vi "Illini Hyperloop GUI v2.9.vi"() -> ()   [LabVIEW 2015]
uses:
  <vilib>/ErrorRing/Error Ring.xnode
  BlockDiagramControlEnum.ctl
  <vilib>/robotics/Controls/Attitude Indicator/Attitude Indicator.xctl
  CommunicationStatus.ctl
  StageEnum.ctl
panel:
  in  "Client Closed 2":string="The client VI closed the connection."
  out "Braking Force":dbl
  out "Braking Force Chart":dbl(slide) caption="Braking Force (N)" scale=0.0..10000.0
  out "Current 6":dbl[unit] caption="Current"
  out "Voltage 6":dbl[unit] caption="Voltage"
  out "RPM 6":dbl[unit] caption="RPM"
  out "Current 5":dbl[unit] caption="Current"
  out "Voltage 5":dbl[unit] caption="Voltage"
  out "RPM 5":dbl[unit] caption="RPM"
  out "Current 4":dbl[unit] caption="Current"
  out "Voltage 4":dbl[unit] caption="Voltage"
  out "RPM 4":dbl[unit] caption="RPM"
  out "Current 3":dbl[unit] caption="Current"
  out "Voltage 3":dbl[unit] caption="Voltage"
  out "RPM 3":dbl[unit] caption="RPM"
  out "Current 2":dbl[unit] caption="Current"
  out "Voltage 2":dbl[unit] caption="Voltage"
  out "RPM 2":dbl[unit] caption="RPM"
  out "Current 1":dbl[unit] caption="Current"
  out "Voltage 1":dbl[unit] caption="Voltage"
  out "RPM 1":dbl[unit] caption="RPM"
  out "Flight Time":string
  out "Attitude Indicator":cluster{"Roll":dbl, "Pitch":dbl}(xcontrol)
  out "Yaw":dbl(knob) scale=-20.0..20.0
  out "RPM Gauge 6":dbl(knob) scale=0.0..2000.0
  out "RPM Gauge 5":dbl(knob) scale=0.0..2000.0
  out "RPM Gauge 4":dbl(knob) scale=0.0..2000.0
  out "RPM Gauge 3":dbl(knob) scale=0.0..2000.0
  out "RPM Gauge 2":dbl(knob) scale=0.0..2000.0
  out "RPM Gauge 1":dbl(knob) scale=0.0..2000.0
  out "Cabin Pressure":dbl format="%#.3g"
  out "Cabin Pressure (psi)":dbl(graph)
  out "Stage":T1
  out "Communication Status":T2
  out "Levitation Height":dbl[unit]
  out "Computing:":dbl format="%#.2g"
  out "Low Battery":dbl format="%#.2g"
  out "High Battery:":dbl format="%#.2g"
  out "Battery 3":dbl(slide) scale=0.0..100.0
  out "Battery 2":dbl(slide) scale=0.0..100.0
  out "Battery 1":dbl(slide) scale=0.0..100.0
  out "Z acceleration":dbl
  out "Y acceleration":dbl
  out "X acceleration":dbl
  out "Z velocity":dbl
  out "Y velocity":dbl
  out "X velocity":dbl
  out "Z position":dbl
  out "Y position":dbl
  out "X position":dbl
  out "Position (m)":dbl(slide) scale=0.0..2490.0
  out "Checkmark":u16(ring)
  out "Velocity (m/s)":dbl(graph)
  in  "EMERGENCY BRAKE":bool
  in  "Functional Test Tab Control":T3(tab)
  out "Functional Test A Data":string caption="Data:"
  in  "Functional Test 1":bool caption="Boolean"
  out "Functional Test B Data":string caption="Data:"
  in  "Functional Test 2":bool caption="Boolean"
  out "Functional Test C Data":string caption="Data:"
  in  "Functional Test 3":bool caption="Boolean"
  in  "Functional Test 4":bool caption="Boolean"
  out "Functional Test D Data":string caption="Data:"
  in  "Client Closed":string="The client VI closed the connection."
  out "Data out":string
  out "remote address":string
  out "remote port":u16
  in  "Prepare for Launch":bool caption="Boolean"
  in  "Stop Program":bool
  out "Temp 2:":dbl format="%.2g"
  out "Temp 1:":dbl format="%.2g"
  out "Temperature (K)":dbl[](graph)
  out "Acceleration Chart":dbl(graph)
  # "Illini Hyperloop"
  # "Arx Pax"
  # "Front"
  # "Attitude"
  # "Acceleration (m/s/s)"
  # "Battery Levels (%)"
  # "More battery?????"
  # "Functional Test A: Power Up and Communication"
  # "Functional Test B: Levitation"
  # "Functional Test C: Communication Inside Tube"
  # "Functional Test D: Internal power and Levitation"
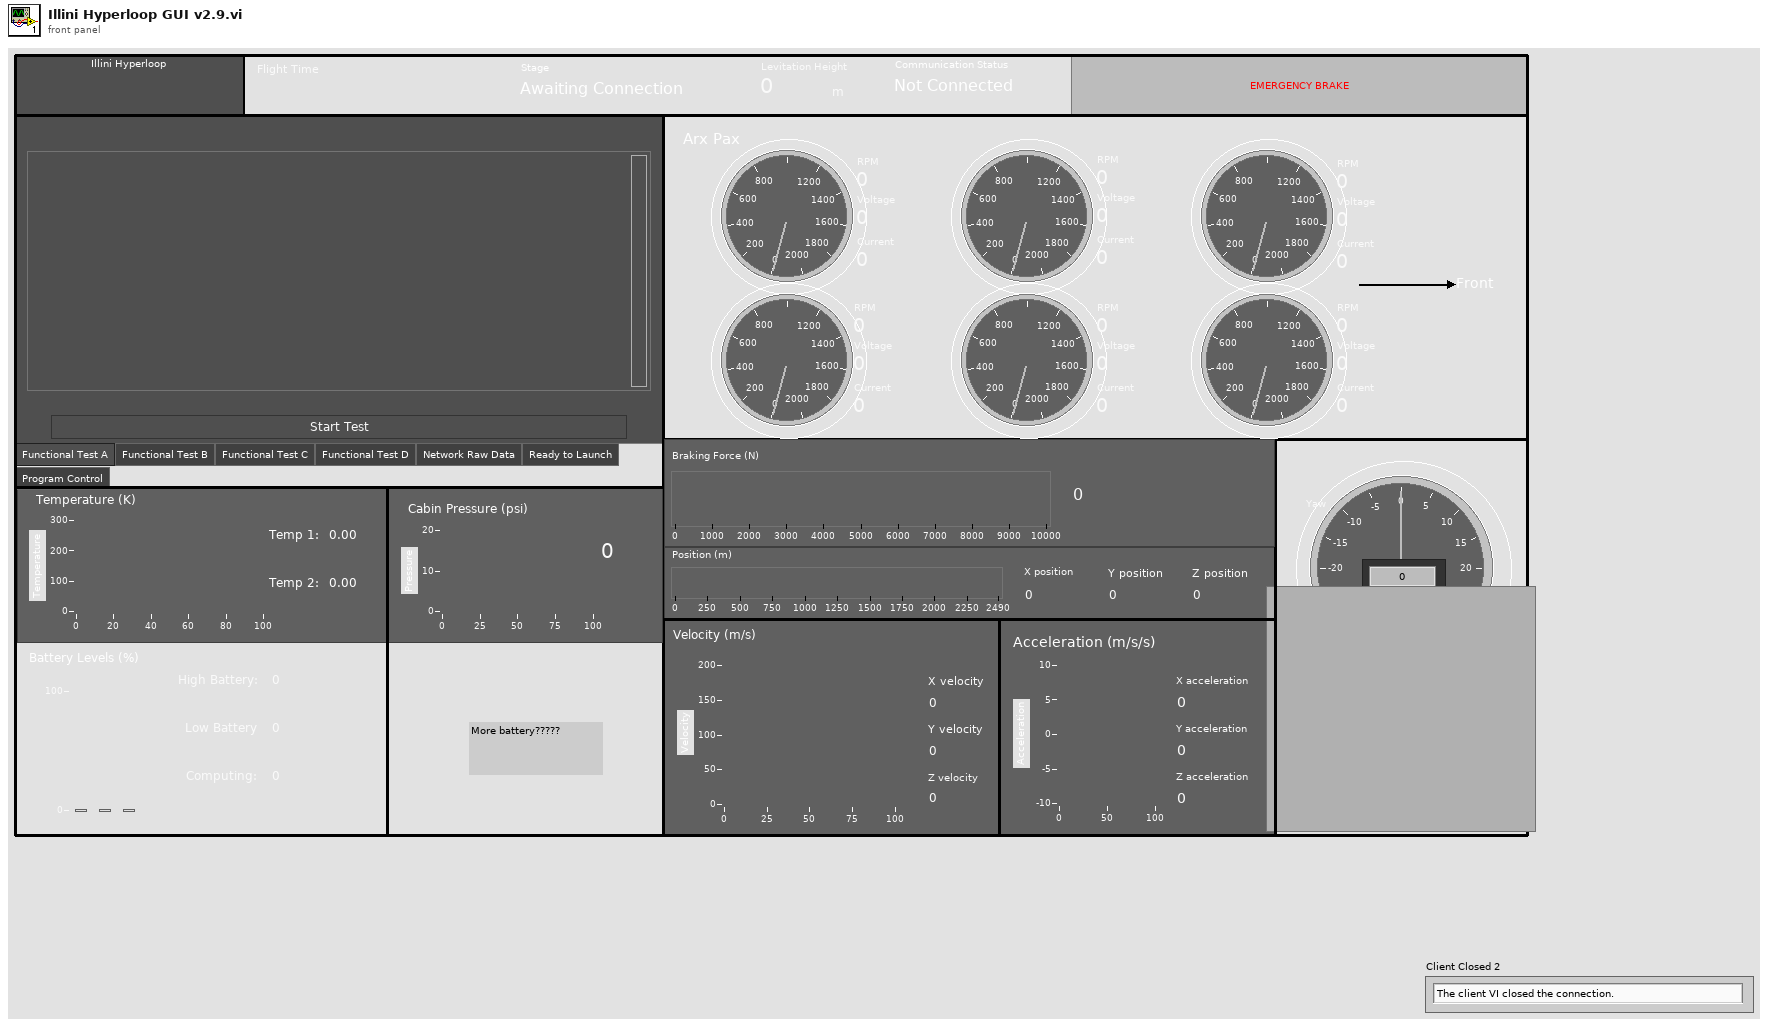
[diagram p1: front panel]
types:
  T1 = typedef "StageEnum.ctl" = enum16{"Awaiting Connection", "TEST Comms", "TEST Lev", "TEST Inside Comms", "TEST Internal Power", "Ready to Launch", "Acceleration", "Coast", "Brake"}
  T2 = typedef "CommunicationStatus.ctl" = enum16{"Not Connected", "Connected", "Disconnected"}
  T3 = enum32{"Functional Test A", "Functional Test B", "Functional Test C", "Functional Test D", "Network Raw Data", "Ready to Launch", "Program Control"}
  T4 = typedef "BlockDiagramControlEnum.ctl" = enum16{"Not Connected", "Disconnected", "Functional Test A", "Functional Test B", "Functional Test C", "Functional Test D", "Flight"}
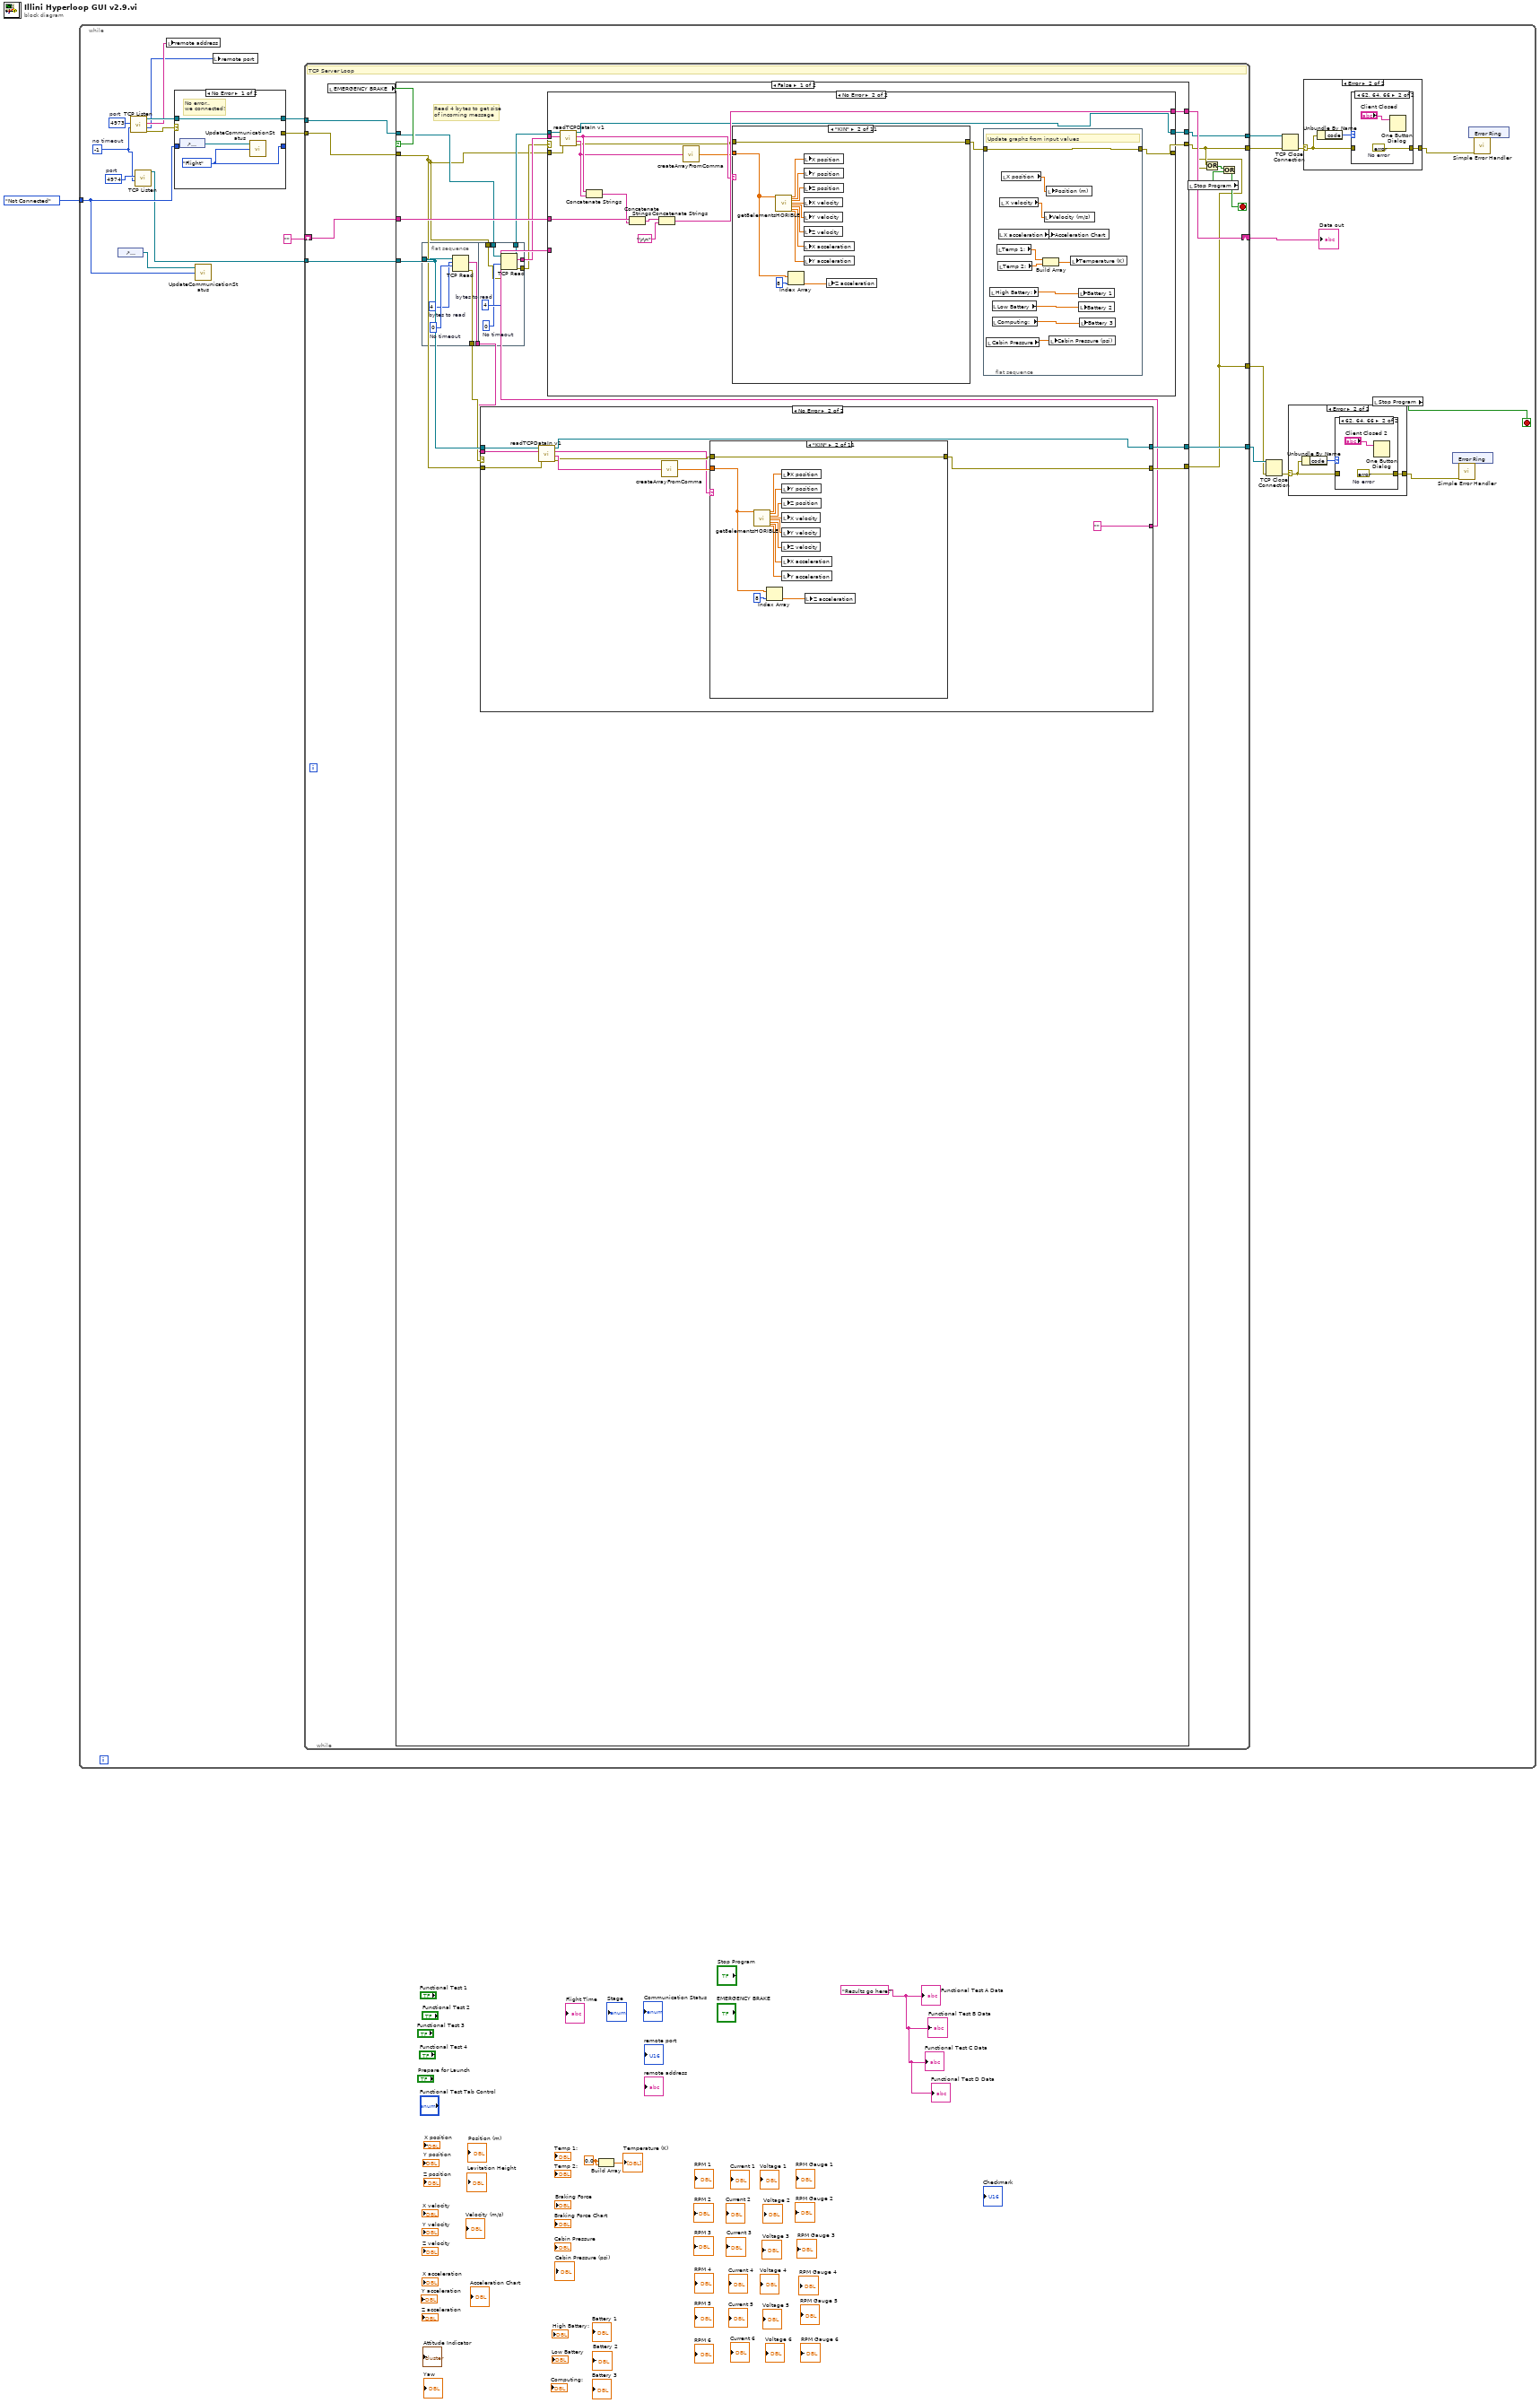
[diagram p0: block diagram]
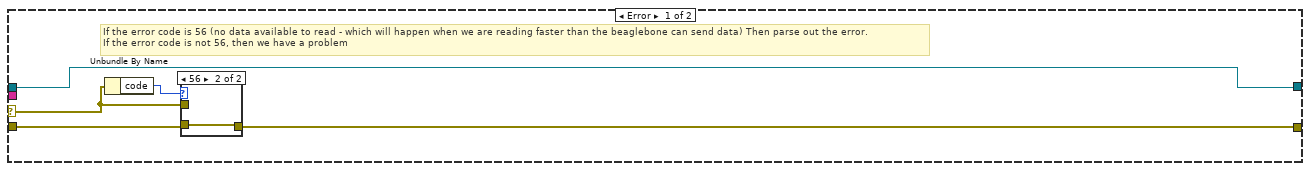
[diagram p7: hidden frame]
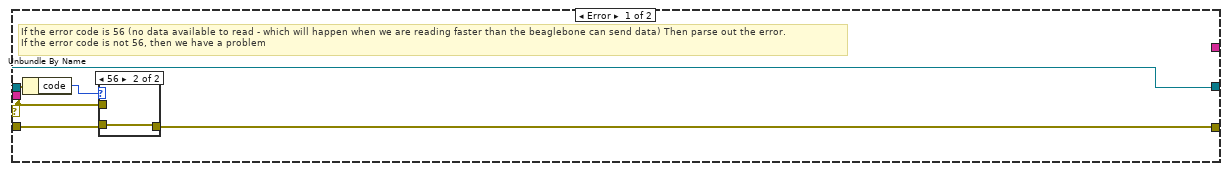
[diagram p19: hidden frame]
diagram:
  w2 = 0.0 ("element")
  w4 = "Results go here!" ("Functional Test 1 Data")
  n1 = while {
    tunnel: BlockDiagramControlEnum."Not Connected" -> [w12]
    stop <- w20 stop-if-true
    w11 = u16 4974  # port
    w25 = u16 4973  # port
    w10 = -1  # no timeout
    n2 = control-ref of="Communication Status"() -> (w13:refnum<vi>)
    n3 = call <vilib>:"TCP Listen.vi"("timeout ms (wait forever: -1)"=w10, "port"=w25) -> ("error out"=w17:errorcluster, "remote port"=w14:u16, "remote address"=w15:string, "connection ID"=w19:refnum<k5>)  [unwired: 5 in, 1 out]
    n4 = call <vilib>:"TCP Listen.vi"("timeout ms (wait forever: -1)"=w10, "port"=w11) -> ("connection ID"=w9:refnum<k5>)  [unwired: 5 in, 4 out]
    n5 = local write "remote address"(w15) -> ()
    n6 = case shown="No Error" w17 {
      selector: w17 -> [_ w40]
      tunnel: w19 -> [w38 w41]
      tunnel: [w38 w41] -> w18
      tunnel: [_ w40] -> w16
      tunnel: w12 -> [_ w39]
      tunnel: [w36 w39] -> _
      frame No Error {
        w36 = BlockDiagramControlEnum."Flight"
        # "No error.. \nwe connected!"
        n7 = control-ref of="Communication Status"() -> (w37:refnum<vi>)
        n8 = call "UpdateCommunicationStatus.vi"("Block Diagram Control Enum"=w36, "Communication Enum Refnum in"=w37) -> ()  [unwired: 1 in]
      }
      frame Error {
      }
    }
    n9 = call "UpdateCommunicationStatus.vi"("Block Diagram Control Enum"=w12, "Communication Enum Refnum in"=w13) -> ()  [unwired: 1 in]
    n10 = local write "remote port"(w14) -> ()
    n11 = while {
      tunnel: w18 -> [w61]
      tunnel: w16 -> [w62]
      shift-right: [w59] -> w23
      shift-left: "" -> [w60]
      tunnel: [w58] -> w22
      tunnel: [w53] -> w21
      tunnel: w9 -> [w54]
      tunnel: [w51] -> w6
      tunnel: [w50] -> w5
      stop <- w55 stop-if-true
      # "TCP Server Loop"
      n12 = local read "EMERGENCY BRAKE"() -> (w57:bool)
      n13 = case shown="False" w57 {
        tunnel: w62 -> [w64 w236]
        tunnel: w61 -> [w68 w235]
        tunnel: [w77 w234] -> w58
        tunnel: [w78 w233] -> w53
        tunnel: w60 -> [w76 _]
        tunnel: [w75 _] -> w59
        tunnel: w54 -> [w74 w232]
        tunnel: [w71 _] -> w50
        tunnel: [w70 w232] -> w51
        frame False {
          # "Read 4 bytes to get size\nof incoming message"
          n14 = flat-sequence {
            tunnel: w74 -> [w81]
            tunnel: [w80] -> w73
            tunnel: [w79] -> w72
            tunnel: w68 -> [w88]
            tunnel: w64 -> [w87]
            tunnel: [w86] -> w67
            tunnel: [w85] -> w66
            tunnel: [w84] -> w65
            frame #0 {
              w82 = 4  # bytes to read
              w83 = 0  # No timeout
              n15 = TCP Read(connection ID=w81, bytes to read=w82, 9:w83) -> (data out=w79:string, error out=w80:errorcluster)  [unwired: 2 in, 1 out]
            }
            frame #1 {
              w90 = 4  # bytes to read
              w89 = 0  # No timeout
              n16 = TCP Read(connection ID=w88, bytes to read=w90, error in (no error)=w87, 9:w89) -> (connection ID out=w86:refnum<k5>, data out=w85:string, error out=w84:errorcluster)  [unwired: 1 in]
            }
          }
          n17 = case shown="No Error" w73 {
            selector: w73 -> [w93 _]
            tunnel: w64 -> [w94 w105]
            tunnel: [w92 w100] -> w71
            tunnel: w74 -> [w91 w106]
            tunnel: [w91 w99] -> w70
            tunnel: w72 -> [_ w107]
            tunnel: [_ ""] -> w69
            frame Error {
              # "If the error code is 56 (no data available to read - which will happen when we are reading faster than the beaglebone can send data) Then parse out the error. \nIf the error code is not 56, then we have a problem"
              n18 = Unbundle By Name(w93) -> ("code"=w95:i32)
              n19 = case shown="56" w95 {
                tunnel: w93 -> [w96 _]
                tunnel: [w96 w97] -> w92
                tunnel: w94 -> [_ w97]
                frame Default {
                }
                frame 56 {
                }
              }
            }
            frame No Error {
              n20 = call "readTCPDataIn v1.vi"("error in (no error)"=w105, "Size of data"=w107, "TCP Network Connection in"=w106) -> ("error out"=w102:errorcluster, "Data"=w104:string, "Operation"=w101:string, "TCP Network Connection out"=w99:refnum<k5>)  [unwired: 5 in]
              n21 = call "createArrayFromComma.vi"("String"=w104) -> ("Array"=w103:dbl[])
              n22 = case shown="\"KIN\"" w101 {
                tunnel: w103 -> [_ w119 _ _ _ _ _ _ _ _ _]
                tunnel: w102 -> [w108 w117 w121 w122 w123 w124 w125 w126 w127 w128 w129]
                tunnel: [w108 w117 w121 w122 w123 w124 w125 w126 w127 w128 w129] -> w100
                frame Default {
                }
                frame "KIN" {
                  n23 = call "get8elementsHORIBLE.vi"("Array"=w119) -> ("Numeric"=w116:dbl, "Numeric 2"=w115:dbl, "Numeric 3"=w114:dbl, "Numeric 4"=w113:dbl, "Numeric 5"=w112:dbl, "Numeric 6"=w111:dbl, "Numeric 7"=w110:dbl, "Numeric 8"=w109:dbl)  [unwired: 19 in]
                  n24 = Index Array(array=w119, index=8) -> (element=w118:dbl)
                  n25 = local write "X position"(w116) -> ()
                  n26 = local write "Y position"(w115) -> ()
                  n27 = local write "Z position"(w114) -> ()
                  n28 = local write "X velocity"(w113) -> ()
                  n29 = local write "Y velocity"(w112) -> ()
                  n30 = local write "Z velocity"(w111) -> ()
                  n31 = local write "X acceleration"(w110) -> ()
                  n32 = local write "Y acceleration"(w109) -> ()
                  n33 = local write "Z acceleration"(w118) -> ()
                }
                frame "ALL" {
                }
                frame "ATT" {
                }
                frame "TMP" {
                }
                frame "BAT" {
                }
                frame "CBP" {
                }
                frame "FTA" {
                }
                frame "FTB" {
                }
                frame "FCC" {
                }
                frame "FCD" {
                }
              }
            }
          }
          n34 = case shown="No Error" w65 {
            selector: w65 -> [w132 _]
            tunnel: w64 -> [w133 w149]
            tunnel: [w131 w137] -> w78
            tunnel: w67 -> [w130 w150]
            tunnel: [w130 w138] -> w77
            tunnel: w66 -> [_ w151]
            tunnel: w76 -> [_ w148]
            tunnel: [_ w144] -> w75
            tunnel: w69 -> [_ _]
            frame Error {
              # "If the error code is 56 (no data available to read - which will happen when we are reading faster than the beaglebone can send data) Then parse out the error. \nIf the error code is not 56, then we have a problem"
              n35 = Unbundle By Name(w132) -> ("code"=w134:i32)
              n36 = case shown="56" w134 {
                tunnel: w132 -> [w135 _]
                tunnel: [w135 w136] -> w131
                tunnel: w133 -> [_ w136]
                frame Default {
                }
                frame 56 {
                }
              }
            }
            frame No Error {
              n37 = call "readTCPDataIn v1.vi"("error in (no error)"=w149, "Size of data"=w151, "TCP Network Connection in"=w150) -> ("error out"=w139:errorcluster, "Data"=w141:string, "Operation"=w143:string, "TCP Network Connection out"=w138:refnum<k5>)  [unwired: 5 in]
              n38 = Concatenate Strings(w143, w141) -> (w142:string)
              n39 = Concatenate Strings(w148, w142) -> (w145:string)
              n40 = Concatenate Strings(w145, "\r\n") -> (w144:string)
              n41 = call "createArrayFromComma.vi"("String"=w141) -> ("Array"=w140:dbl[])
              n42 = case shown="\"KIN\"" w143 {
                tunnel: w140 -> [_ w174 w178 w206 w213 w220 w226 _ _ _ _]
                tunnel: w139 -> [w163 w172 w176 w201 w210 w216 w224 w228 w229 w230 w231]
                tunnel: [w163 w172 w176 w201 w210 w216 w224 w228 w229 w230 w231] -> w147
                frame Default {
                }
                frame "KIN" {
                  n43 = call "get8elementsHORIBLE.vi"("Array"=w174) -> ("Numeric"=w171:dbl, "Numeric 2"=w170:dbl, "Numeric 3"=w169:dbl, "Numeric 4"=w168:dbl, "Numeric 5"=w167:dbl, "Numeric 6"=w166:dbl, "Numeric 7"=w165:dbl, "Numeric 8"=w164:dbl)  [unwired: 19 in]
                  n44 = Index Array(array=w174, index=8) -> (element=w173:dbl)
                  n45 = local write "X position"(w171) -> ()
                  n46 = local write "Y position"(w170) -> ()
                  n47 = local write "Z position"(w169) -> ()
                  n48 = local write "X velocity"(w168) -> ()
                  n49 = local write "Y velocity"(w167) -> ()
                  n50 = local write "Z velocity"(w166) -> ()
                  n51 = local write "X acceleration"(w165) -> ()
                  n52 = local write "Y acceleration"(w164) -> ()
                  n53 = local write "Z acceleration"(w173) -> ()
                }
                frame "ALL" {
                  n54 = call "get8elementsHORIBLE.vi"("Array"=w178) -> ("Numeric"=w198:dbl, "Numeric 2"=w197:dbl, "Numeric 3"=w196:dbl, "Numeric 4"=w195:dbl, "Numeric 5"=w194:dbl, "Numeric 6"=w193:dbl, "Numeric 7"=w192:dbl, "Numeric 8"=w191:dbl)  [unwired: 19 in]
                  n55 = local write "X position"(w198) -> ()
                  n56 = local write "Y position"(w197) -> ()
                  n57 = local write "Z position"(w196) -> ()
                  n58 = local write "X velocity"(w195) -> ()
                  n59 = local write "Y velocity"(w194) -> ()
                  n60 = local write "Z velocity"(w193) -> ()
                  n61 = local write "X acceleration"(w192) -> ()
                  n62 = local write "Y acceleration"(w191) -> ()
                  n63 = Index Array(array=w178, index=17) -> (element=w177:dbl)
                  n64 = local write "Cabin Pressure"(w177) -> ()
                  n65 = Array Subset(array=w178, index=9) -> (w188:dbl[])  [unwired: 1 in]
                  n66 = call "get8elementsHORIBLE.vi"("Array"=w188) -> ("Numeric"=w187:dbl, "Numeric 2"=w186:dbl, "Numeric 3"=w185:dbl, "Numeric 4"=w184:dbl, "Numeric 5"=w183:dbl, "Numeric 6"=w182:dbl, "Numeric 7"=w181:dbl, "Numeric 8"=w180:dbl)  [unwired: 19 in]
                  n67 = Index Array(array=w178, index=8) -> (element=w199:dbl)
                  n68 = local write "High Battery:"(w182) -> ()
                  n69 = local write "Computing:"(w180) -> ()
                  n70 = local write "Low Battery"(w181) -> ()
                  n71 = local write "Yaw"(w185) -> ()
                  n72 = local write "Temp 1:"(w184) -> ()
                  n73 = local write "Temp 2:"(w183) -> ()
                  n74 = Bundle("Numeric"=w187, "Numeric 2"=w186) -> (w190:cluster{"Numeric":dbl, "Numeric 2":dbl})  [unwired: 1 in]
                  n75 = local write "Z acceleration"(w199) -> ()
                  n76 = local write "Attitude Indicator"(w190) -> ()
                }
                frame "ATT" {
                  n77 = Index Array(array=w206, index=0) -> (element=w205:dbl)
                  n78 = Index Array(array=w206, index=1) -> (element=w204:dbl)
                  n79 = Index Array(array=w206, index=2) -> (element=w202:dbl)
                  n80 = Bundle(w205, w204) -> (w203:cluster{dbl, dbl})  [unwired: 1 in]
                  n81 = local write "Yaw"(w202) -> ()
                  n82 = local write "Attitude Indicator"(w203) -> ()
                }
                frame "TMP" {
                  n83 = Index Array(array=w213, index=0) -> (element=w212:dbl)
                  n84 = Index Array(array=w213, index=1) -> (element=w211:dbl)
                  n85 = local write "Temp 1:"(w212) -> ()
                  n86 = local write "Temp 2:"(w211) -> ()
                }
                frame "BAT" {
                  n87 = Index Array(array=w220, index=0) -> (element=w219:dbl)
                  n88 = Index Array(array=w220, index=1) -> (element=w218:dbl)
                  n89 = Index Array(array=w220, index=2) -> (element=w217:dbl)
                  n90 = local write "High Battery:"(w219) -> ()
                  n91 = local write "Computing:"(w217) -> ()
                  n92 = local write "Low Battery"(w218) -> ()
                }
                frame "CBP" {
                  n93 = Index Array(array=w226, index=0) -> (element=w225:dbl)
                  n94 = local write "Cabin Pressure"(w225) -> ()
                }
                frame "FTA" {
                }
                frame "FTB" {
                }
                frame "FCC" {
                }
                frame "FCD" {
                }
              }
              n95 = flat-sequence {
                tunnel: w147 -> [w159]
                tunnel: [w159] -> w137
                frame #0 {
                  # "Update graphs from input values"
                  n96 = local read "Cabin Pressure"() -> (w155:dbl)
                  n97 = local read "High Battery:"() -> (w158:dbl)
                  n98 = local read "Low Battery"() -> (w157:dbl)
                  n99 = local read "Computing:"() -> (w156:dbl)
                  n100 = local read "Temp 1:"() -> (w154:dbl)
                  n101 = local read "Temp 2:"() -> (w153:dbl)
                  n102 = local read "X acceleration"() -> (w160:dbl)
                  n103 = local read "X velocity"() -> (w161:dbl)
                  n104 = local read "X position"() -> (w162:dbl)
                  n105 = Build Array(w154, w153) -> (w152:dbl[])
                  n106 = local write "Velocity (m/s)"(w161) -> ()
                  n107 = local write "Acceleration Chart"(w160) -> ()
                  n108 = local write "Position (m)"(w162) -> ()
                  n109 = local write "Cabin Pressure (psi)"(w155) -> ()
                  n110 = local write "Temperature (K)"(w152) -> ()
                  n111 = local write "Battery 1"(w158) -> ()
                  n112 = local write "Battery 2"(w157) -> ()
                  n113 = local write "Battery 3"(w156) -> ()
                }
              }
            }
          }
        }
        frame True {
          n114 = TCP Write(connection ID=w235, data in="STOP!STOP", error in (no error)=w236) -> (connection ID out=w234:refnum<k5>, error out=w233:errorcluster)  [unwired: 1 in, 1 out]
        }
      }
      n115 = Wait (ms)(milliseconds to wait=u32 0) -> ()  [unwired: 1 out]
      n116 = local read "Stop Program"() -> (w56:bool)
      n117 = Or(x=w53, y=w50) -> (x .or. y?=w52:bool)
      n118 = Or(x=w52, y=w56) -> (x .or. y?=w55:bool)
    }
    "Data out" <- w23
    n119 = TCP Close Connection(connection ID=w6, error in (no error)=w5) -> (error out=w8:errorcluster)  [unwired: 2 out]
    n120 = TCP Close Connection(connection ID=w22, error in (no error)=w21) -> (error out=w27:errorcluster)  [unwired: 2 out]
    n121 = case shown="Error" w8 {
      selector: w8 -> [w29 w31]
      tunnel: [w29 w30] -> w7
      frame No Error {
      }
      frame Error {
        n122 = Unbundle By Name(w31) -> ("code"=w32:i32)
        n123 = case shown="62, 64, 66" w32 {
          tunnel: w31 -> [w33 _]
          tunnel: [w33 w35] -> w30
          frame Default {
          }
          frame 62, 64, 66 {
            w35 = errorcluster {"status"=FALSE, "code"=0, "source"=""}  # No error
            n124 = One Button Dialog(message="Client Closed 2") -> ()  [unwired: 1 in, 1 out]
          }
        }
      }
    }
    n125 = case shown="Error" w27 {
      selector: w27 -> [w43 w45]
      tunnel: [w43 w44] -> w26
      frame No Error {
      }
      frame Error {
        n126 = Unbundle By Name(w45) -> ("code"=w46:i32)
        n127 = case shown="62, 64, 66" w46 {
          tunnel: w45 -> [w47 _]
          tunnel: [w47 w49] -> w44
          frame Default {
          }
          frame 62, 64, 66 {
            w49 = errorcluster {"status"=FALSE, "code"=0, "source"=""}  # No error
            n128 = One Button Dialog(message="Client Closed") -> ()  [unwired: 1 in, 1 out]
          }
        }
      }
    }
    n129 = local read "Stop Program"() -> (w20:bool)
    n130 = xnode "Error Ring"() -> ()  [unwired: 1 out]
    n131 = call <vilib>:"Simple Error Handler.vi"("error in (no error)"=w7) -> ()  [unwired: 1 in, 8 out]
    n132 = xnode "Error Ring"() -> ()  [unwired: 1 out]
    n133 = call <vilib>:"Simple Error Handler.vi"("error in (no error)"=w26) -> ()  [unwired: 1 in, 8 out]
  }
  n134 = Build Array(w2, w2) -> (→"Temperature (K)":dbl[])
  "Functional Test A Data" <- w4
  "Functional Test B Data" <- w4
  "Functional Test C Data" <- w4
  "Functional Test D Data" <- w4
